vi "SC2250 Session Map.vi"(0 "Instrument name":string, 1 "Action":T1, 5 "sc2250 session in":refnum<k15>) -> (4 "sc2250 session":refnum<k15>, 6 "sc2250 session not found / already included":bool, 10 "sc2250 sessions":refnum<k15>[](array[refnum]))   [LabVIEW 2023, in "RFFixtureCharact.RFPM.lvlib" / "SG SC2250 Path Group.lvclass"]
uses:
  SG SC2250 Path Group.lvclass
  Common/Data Cache/Type Definitions/Dictionary Operation.ctl
  Common/RFCalAndFixtureCharact.Common.lvlib
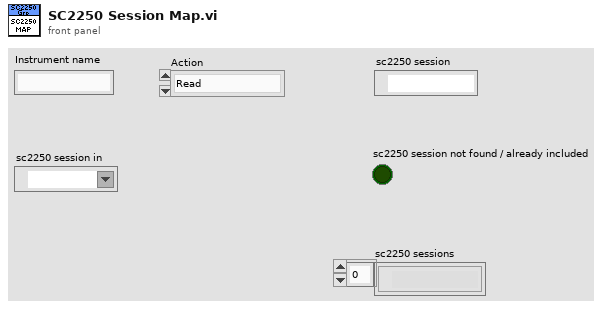
[diagram p1: front panel]
types:
  T1 = typedef "RFCalAndFixtureCharact.Common.lvlib/Dictionary Operation.ctl" = enum16{"Read", "Insert", "Remove", "Clear", "Get All", "Update"}
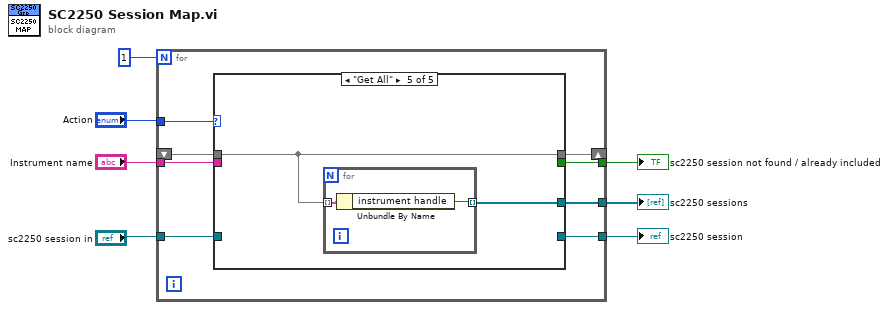
[diagram p0: block diagram]
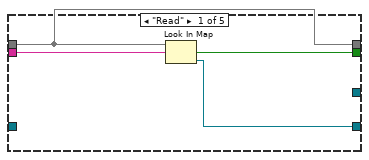
[diagram p2: hidden frame]
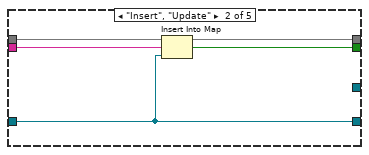
[diagram p3: hidden frame]
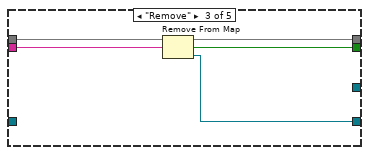
[diagram p4: hidden frame]
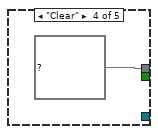
[diagram p5: hidden frame]
diagram:
  n1 = for {
    N: 1 -> [_]
    tunnel: "Action" -> [w15]
    tunnel: "Instrument name" -> [w14]
    tunnel: [w13] -> w5
    tunnel: [w12] -> w4
    shift-right: [w10] -> _
    shift-left: _ -> [w11]
    tunnel: "sc2250 session in" -> [w9]
    tunnel: [w8] -> w2
    n2 = case shown="\"Get All\"" w15 {
      tunnel: w14 -> [w19 w24 w27 _ _]
      tunnel: w11 -> [w17 w23 w28 _ w32]
      tunnel: [w18 w22 w29 _ _] -> w13
      tunnel: [w16 w20 w26 _ _] -> w12
      tunnel: [w17 w21 w25 map{string, refnum<k15>} {} ("map") w32] -> w10
      tunnel: w9 -> [_ w20 _ _ _]
      tunnel: [_ _ _ _ w31] -> w8
      frame "Read" {
        n3 = Look In Map(map=w17, key=w19) -> (key not found?=w18:bool, value=w16:refnum<k15>)  [unwired: 1 in]
      }
      frame "Insert", "Update" {
        n4 = Insert Into Map(map in=w23, key=w24, value=w20) -> (map out=w21:map{string, refnum<k15>}, key already included?=w22:bool)  [unwired: 1 out]
      }
      frame "Remove" {
        n5 = Remove From Map(10:w27, 11:w28) -> (1:w26:refnum<k15>, 2:w29:bool, 3:w25:map{string, refnum<k15>})
      }
      frame "Clear" {
      }
      frame "Get All" {
        n6 = for {
          tunnel: w32 -> [w34] mode=indexing
          tunnel: [w33] -> w31 mode=indexing
          n7 = Unbundle By Name(w34) -> ("instrument handle"=w33:refnum<k15>)
        }
      }
    }
  }
  "sc2250 session not found / already included" <- w5
  "sc2250 sessions" <- w2
  "sc2250 session" <- w4
